vi "Station.Execution.vi"() -> ()   [LabVIEW 2015]
uses:
  Types/Main.StateVariables.ctl
  <vilib>/Utility/miscctls.llb/LVPositionTypeDef.ctl
  Types/Execute.UserEventRefs.ctl
  <vilib>/NI Veristand/Execution/Workspace/SystemStateRegEventRef.ctl
  <vilib>/NI Veristand/Execution/Workspace/Target State Info.ctl
  <vilib>/NI Veristand/Execution/Workspace/Target State.ctl
  <vilib>/NI Veristand/Execution/WaveformStreaming/Waveform Data Watcher Event Data (DBL).ctl
  <vilib>/NI Veristand/Execution/WaveformStreaming/WaveformStreamSpecification.ctl
  <vilib>/NI Veristand/Execution/Workspace/SystemStateEventRef.ctl
  <vilib>/NI Veristand/Execution/Workspace/WorkspaceAPI.ctl
  Types/UI.Object.ctl
  Types/Waveforms.Info.ctl
  <vilib>/NI Veristand/Execution/WaveformStreaming/Registered Waveform Streams Data Event Refnum (DBL).ctl
  <vilib>/NI Veristand/Execution/WaveformStreaming/WaveformDataWatcherDBL.ctl
  <vilib>/NI Veristand/Execution/WaveformStreaming/WaveformStreamingAPI.ctl
  <vilib>/NI/AMC/Read Termination Message.vi
  <vilib>/NI/AMC/Create Single Message.vi
  <vilib>/NI/AMC/Update Message Routing Info.vi
  <vilib>/NI/AMC/Create Multiple Messages.vi
  <vilib>/NI/AMC/Globals.vi
  <vilib>/NI/AMC/Send Message.vi
  NationalInstruments.VeriStand.ClientAPI
  <vilib>/NI Veristand/Execution/Workspace/NI_VS Workspace ExecutionAPI.lvlib
  <vilib>/NI/AMC/AMC.lvlib
  <vilib>/NI Veristand/Execution/WaveformStreaming/NI_VS Waveform Streaming Interface.lvlib
panel:
  in  "Tabs":string[](array[string])=["CAN.Fault Status", "CAN.IDH", "CAN.IDL", "CAN.LIN", "CAN.ODH", "CAN.ODL", "CAN.OPH", "DAQ.IDH", "DAQ.IDL", "DAQ.ODH", "DAQ.ODL", "DAQ.OPH"]
  in  "Station.ID":string="DUT1"
  out "Station ID":string="Station 1"
  in  "NIVS.Gateway IP Address":string="localhost"
  in  "NIVS.Workspace Event":refnum<event-registration>
  in  "ToolTab":enum32{"Enable", "Disable"}(tab)
  in  "Back":bool
  in  "Next":bool
  in  "Displays":enum32{"Default", "OSCOPE"}(tab)
  out "Table":string[][](table) caption="DMM"
  in  "Show Chart":bool
  out "Chart":dbl[][](graph)
  in  "Chart.Select":bool
  in  "Waveform.Select":bool
  out "Waveform.Graph":waveform(dbl)[](graph)
  in  "Waveform.Groups":u8(ring) items=["", "All"]
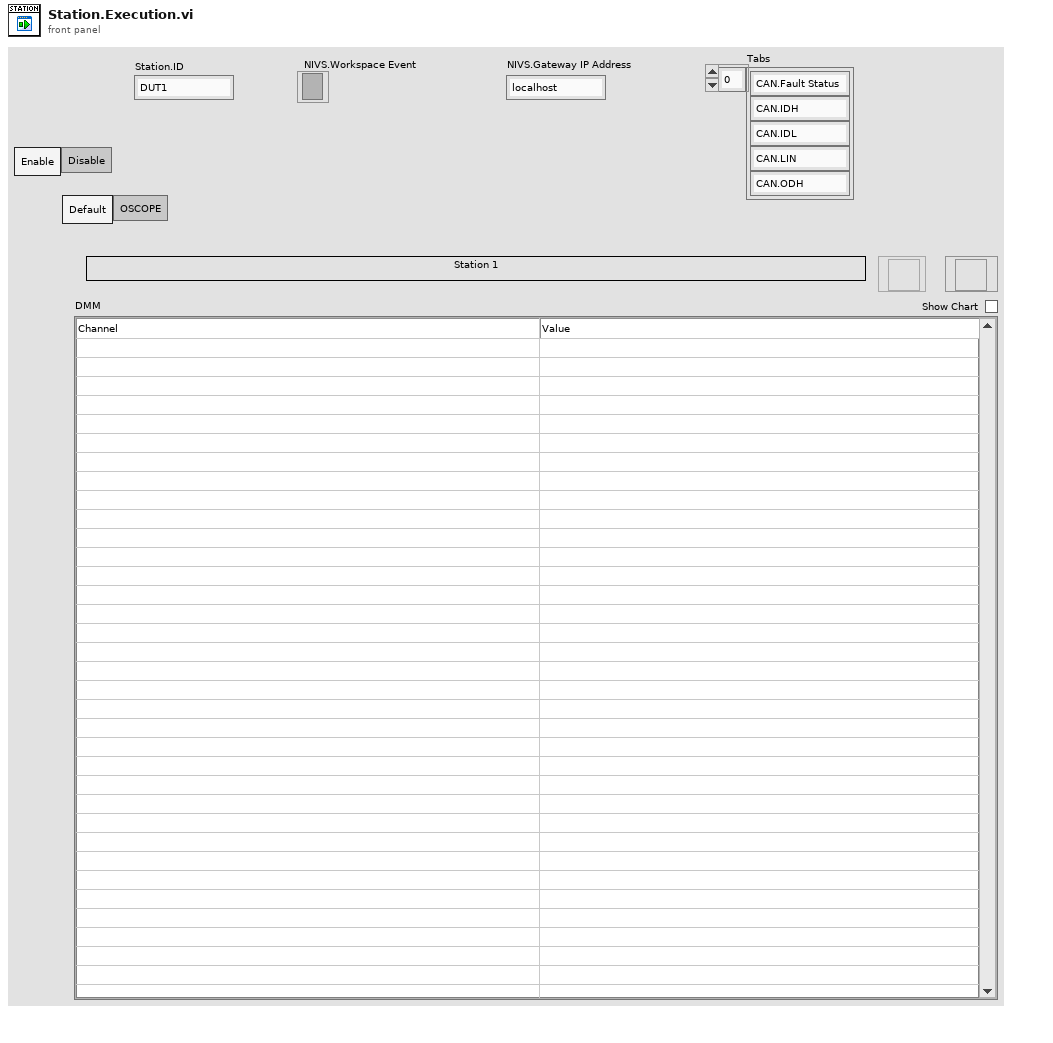
[diagram p1: front panel]
types:
  T1 = typedef "UI.Object.ctl" = cluster{"Name":string, "Paths":string[], "Names":string[], "Found?":bool}
  T2 = typedef "Main.StateVariables.ctl" = cluster{"Chart.Legend":T3, "Chart.Select":refnum<vi>, "Chart.Size":i32, "NIVS.Deployed":bool, "NIVS.Events":T4, "NIVS.GatewayIPAddress":string, "NIVS.SystemDefinitionFile":path, "NIVS.SystemStateRefs":T6, "NIVS.WorkspaceManager":T7, "NIVS.Open":bool, "Page.Index":u32, "Station.ID":string, "UI.Back":refnum<vi>, "UI.Next":refnum<vi>, "UI.Displays":refnum<vi>, "UI.ToolTab":refnum<vi>, "UI.Chart":refnum<vi>, "UI.ShowChart":bool, "UI.Table":refnum<vi>, "UI.Pages":T1[], "VI.Ref":refnum<vi>, "Waveform.Groups":refnum<vi>, "Waveform.Select":refnum<vi>, "Waveform.Graph":refnum<vi>, "Waveforms.Info":T8[], "Waveforms":cluster{"Refs":T9[], "Event.Refs":T10, "Streaming.Ref":T12}, "Waveforms.Reset":bool, "Waveforms.Size":i32, "Waveform.Legend":T3}
  T3 = typedef "LVPositionTypeDef.ctl" = cluster{"Left":i32, "Top":i32}
  T4 = typedef "Execute.UserEventRefs.ctl" = cluster{"SystemChangeEvent":T5, "WorkspaceEvent":refnum<event-registration>, "WaveformEvent":refnum<event-registration>}
  T5 = typedef "NI_VS Workspace ExecutionAPI.lvlib/SystemStateRegEventRef.ctl" = refnum<event-registration>
  T6 = typedef "NI_VS Workspace ExecutionAPI.lvlib/SystemStateEventRef.ctl" = cluster{"CustDatRef":refnum<user-event>, "EvtRef":refnum<k27>, "Target State User Event":refnum<user-event>}
  T7 = typedef "NI_VS Workspace ExecutionAPI.lvlib/WorkspaceAPI.ctl" = refnum<k24>
  T8 = typedef "Waveforms.Info.ctl" = cluster{"Name":string, "Path":string}
  T9 = typedef "NI_VS Waveform Streaming Interface.lvlib/WaveformStreamSpecification.ctl" = refnum<k24>
  T10 = typedef "NI_VS Waveform Streaming Interface.lvlib/Registered Waveform Streams Data Event Refnum (DBL).ctl" = cluster{"Callback Refnum":refnum<k27>, "Data Event":refnum<user-event>, "Event Refnum":refnum<event-registration>, "WaveformDataWatcherDBL":T11}
  T11 = typedef "NI_VS Waveform Streaming Interface.lvlib/WaveformDataWatcherDBL.ctl" = refnum<k24>
  T12 = typedef "NI_VS Waveform Streaming Interface.lvlib/WaveformStreamingAPI.ctl" = refnum<k24>
  T13 = typedef "AMC.lvlib/Message Queue.ctl" = refnum<queue>
  T14 = cluster{"Waveform.Refs":T9[], "WaveformStreaming.Event.Refs":T10, "WaveformStreaming.Ref":T12}
  T15 = typedef "AMC.lvlib/Message.ctl" = cluster{"name":string, "value":string, "attributes":T16, "receiver host":string, "receiver process":string, "source host":string, "source process":string, "priority message":bool, "acknowledge message":bool}
  T16 = typedef "Tools_KeyedArray.lvlib/KeyedArray.ctl" = cluster{"keys":string[], "values":string[]}
  T17 = typedef "LVPoint32TypeDef.ctl" = cluster{"Horizontal":i32, "Vertical":i32}
  T18 = cluster{"Refs":T9[], "Event.Refs":T10, "Streaming.Ref":T12}
  T19 = typedef "NI_VS Workspace ExecutionAPI.lvlib/SystemState.ctl" = u8
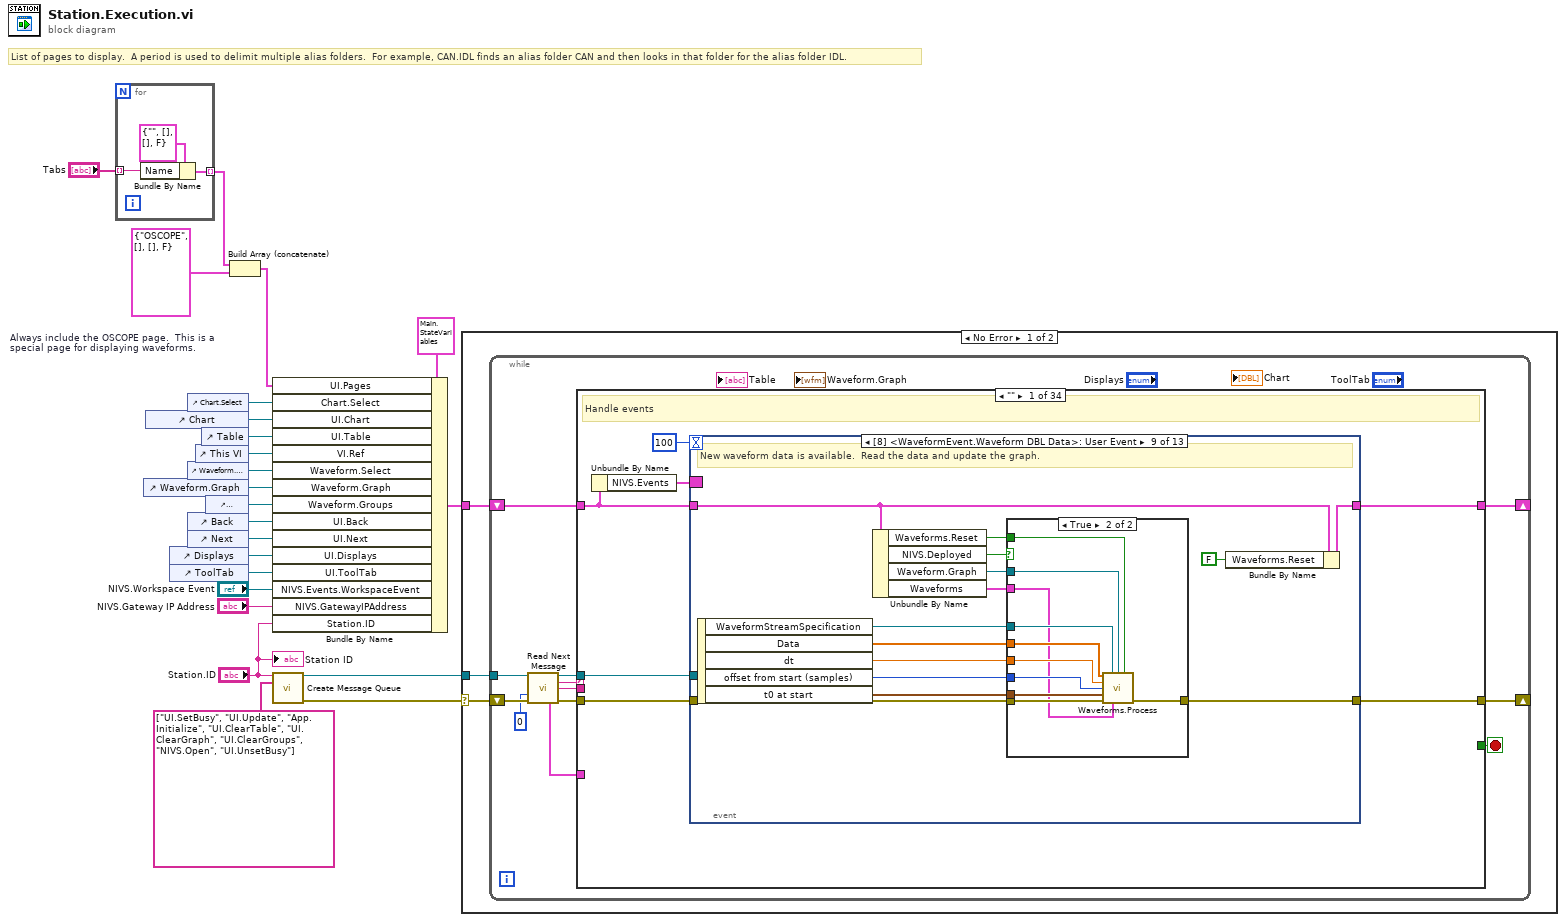
[diagram p0: block diagram]
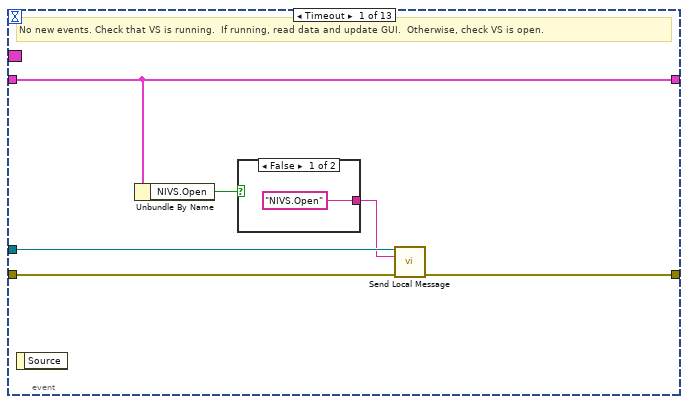
[diagram p2: hidden frame]
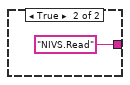
[diagram p3: hidden frame]
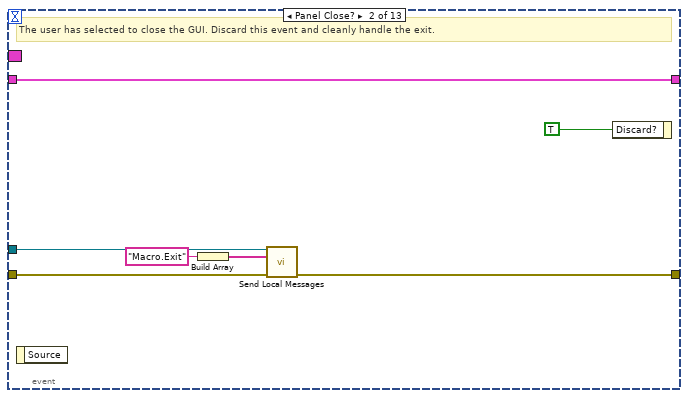
[diagram p4: hidden frame]
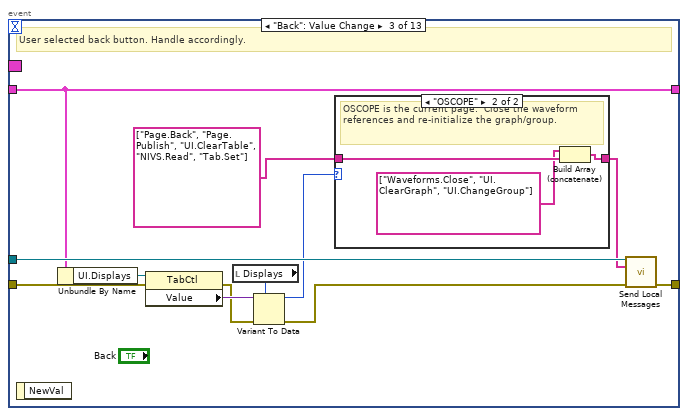
[diagram p5: hidden frame]
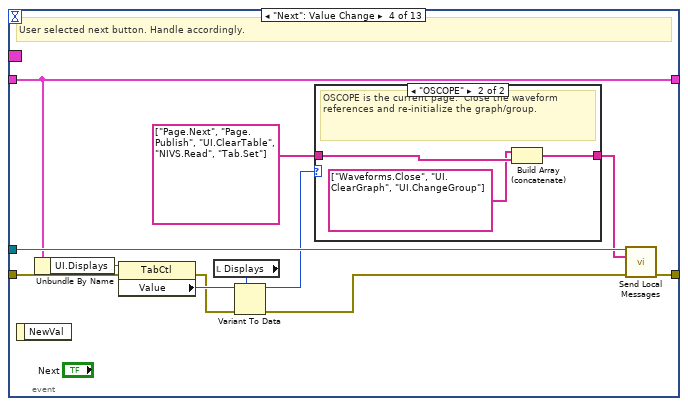
[diagram p7: hidden frame]
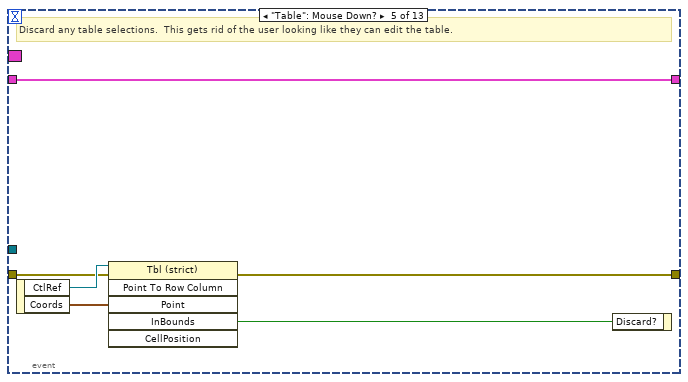
[diagram p9: hidden frame]
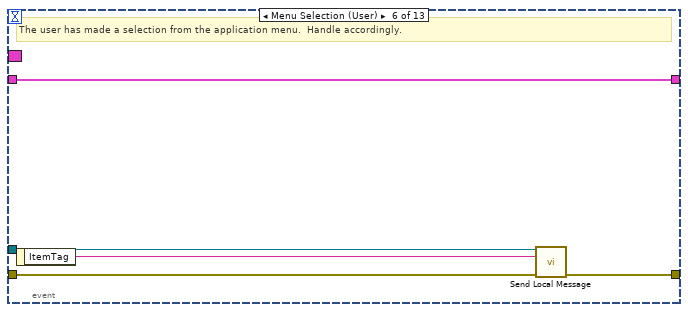
[diagram p10: hidden frame]
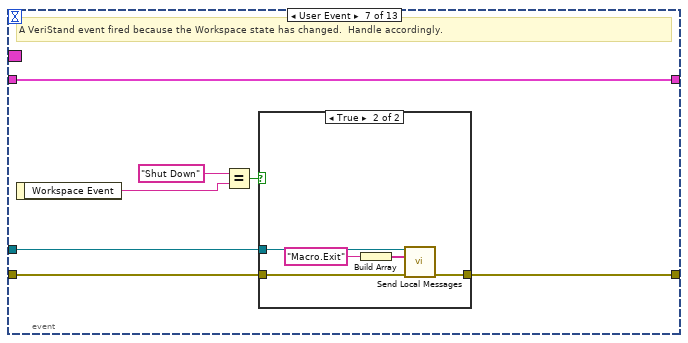
[diagram p11: hidden frame]
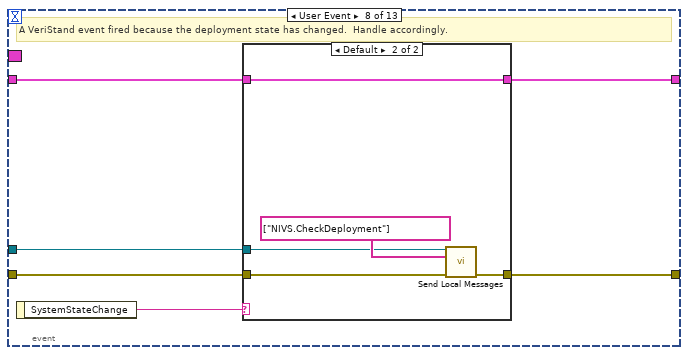
[diagram p13: hidden frame]
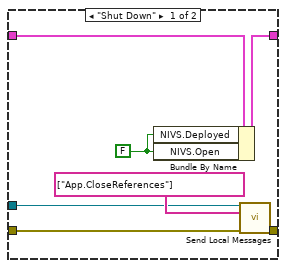
[diagram p14: hidden frame]
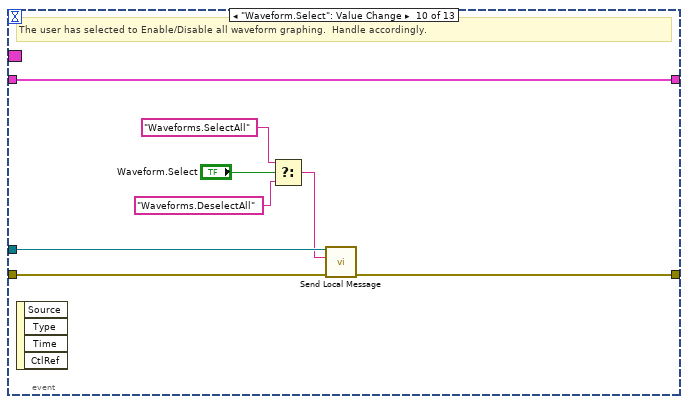
[diagram p16: hidden frame]
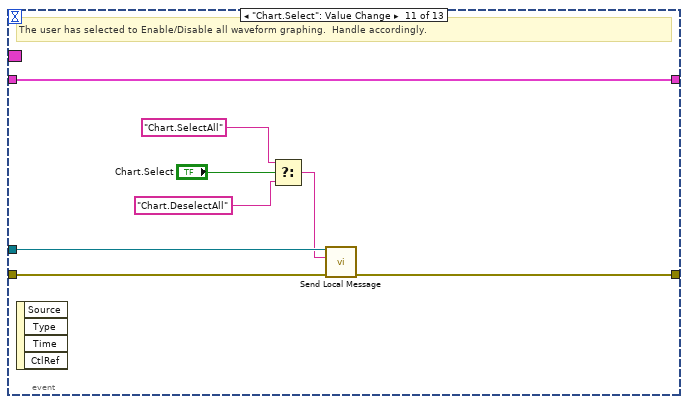
[diagram p17: hidden frame]
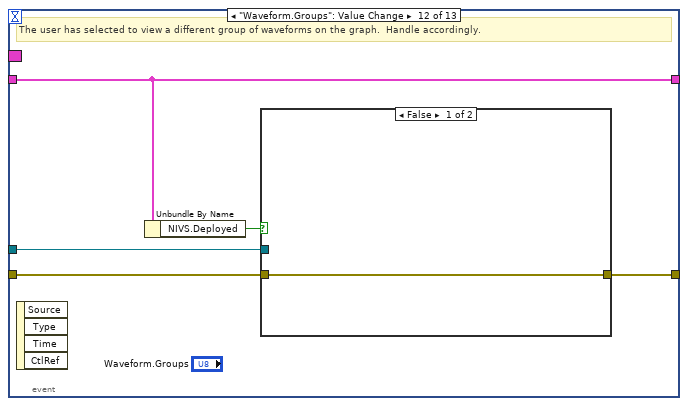
[diagram p18: hidden frame]
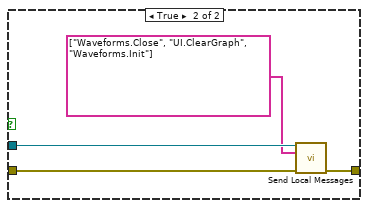
[diagram p19: hidden frame]
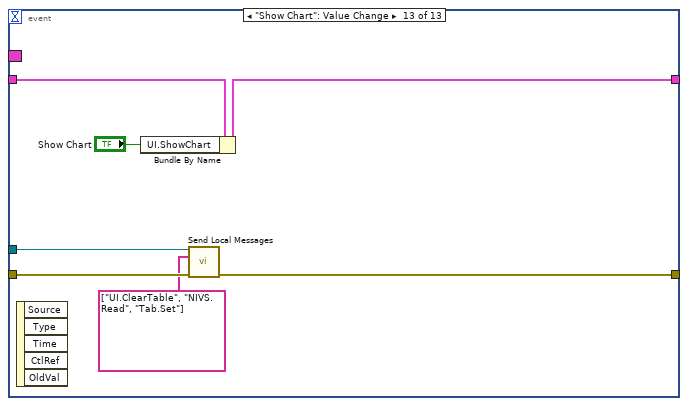
[diagram p20: hidden frame]
diagram:
  w5 = T1 {"Name"="OSCOPE", "Paths"=[], "Names"=[], "Found?"=FALSE}  # Always include the OSCOPE page.  This is a special page for displaying waveforms.
  # "List of pages to display.  A period is used to delimit multiple alias folders.  For example, CAN.IDL finds an alias folder CAN and then looks in that folder for the alias folder IDL."
  n1 = for {
    tunnel: "Tabs" -> [w25] mode=indexing
    tunnel: [w24] -> w4 mode=indexing
    n2 = Bundle By Name(cluster=T1 {"Name"="", "Paths"=[], "Names"=[], "Found?"=FALSE} ("Table"), "Name"=w25) -> (w24:T1)
  }
  n3 = control-ref of="Waveform.Graph"() -> (w8:refnum<vi>)
  n4 = control-ref of="Chart"() -> (w2:refnum<vi>)
  n5 = control-ref of="Displays"() -> (w12:refnum<vi>)
  n6 = control-ref of="ToolTab"() -> (w18:refnum<vi>)
  n7 = control-ref of="Chart.Select"() -> (w1:refnum<vi>)
  n8 = control-ref of="Waveform.Select"() -> (w9:refnum<vi>)
  n9 = control-ref of="Back"() -> (w16:refnum<vi>)
  n10 = control-ref of="Next"() -> (w17:refnum<vi>)
  n11 = control-ref of="This VI"() -> (w11:refnum<vi>)
  n12 = control-ref of="Table"() -> (w3:refnum<vi>)
  n13 = control-ref of="Waveform.Groups"() -> (w10:refnum<vi>)
  n14 = Build Array (concatenate)(w4, w5) -> (w6:T1[])
  n15 = Bundle By Name(cluster=T2 {"Chart.Legend"={"Left"=0, "Top"=0}, "Chart.Select"=refnum, "Chart.Size"=0, "NIVS.Deployed"=FALSE, "NIVS.Events"={"SystemChangeEvent"=refnum, "WorkspaceEvent"=refnum, "WaveformEvent"=refnum}, "NIVS.GatewayIPAddress"="", "NIVS.SystemDefinitionFile"=path "", "NIVS.SystemStateRefs"={"CustDatRef"=refnum, "EvtRef"=refnum, "Target State User Event"=refnum}, "NIVS.WorkspaceManager"=refnum, "NIVS.Open"=FALSE, "Page.Index"=0, "Station.ID"="", "UI.Back"=refnum, "UI.Next"=refnum, "UI.Displays"=refnum, "UI.ToolTab"=refnum, "UI.Chart"=refnum, "UI.ShowChart"=FALSE, "UI.Table"=refnum, "UI.Pages"=[], "VI.Ref"=refnum, "Waveform.Groups"=refnum, "Waveform.Select"=refnum, "Waveform.Graph"=refnum, "Waveforms.Info"=[], "Waveforms"={"Refs"=[], "Event.Refs"={"Callback Refnum"=refnum, "Data Event"=refnum, "Event Refnum"=refnum, "WaveformDataWatcherDBL"=refnum}, "Streaming.Ref"=refnum}, "Waveforms.Reset"=FALSE, "Waveforms.Size"=0, "Waveform.Legend"={"Left"=0, "Top"=0}} ("State Variables"), "UI.Pages"=w6, "Chart.Select"=w1, "UI.Chart"=w2, "UI.Table"=w3, "VI.Ref"=w11, "Waveform.Select"=w9, "Waveform.Graph"=w8, "Waveform.Groups"=w10, "UI.Back"=w16, "UI.Next"=w17, "UI.Displays"=w12, "UI.ToolTab"=w18, "NIVS.Events.WorkspaceEvent"="NIVS.Workspace Event", "NIVS.GatewayIPAddress"="NIVS.Gateway IP Address", "Station.ID"="Station.ID") -> (w23:T2)
  n16 = call <vilib>:"Create Message Queue.vi"("message queue name"="Station.ID", "initial message names"=string[] ["UI.SetBusy", "UI.Update", "App.Initialize", "UI.ClearTable", "UI.ClearGraph", "UI.ClearGroups", "NIVS.Open", "UI.UnsetBusy"]) -> ("message queue out"=w20:T13, "error out"=w13:errorcluster)  [unwired: 12 in]
  n17 = case shown="No Error" w13 {
    selector: w13 -> [w27 _]
    tunnel: w23 -> [w28 _]
    tunnel: w20 -> [w29 _]
    frame No Error {
      n18 = while {
        shift-right: [w40] -> _
        shift-left: w28 -> [w41]
        shift-right: [w30] -> _
        shift-left: w27 -> [w39]
        tunnel: w29 -> [w37]
        stop <- w38 stop-if-true
        n19 = call <vilib>:"Read Next Message.vi"("message queue in"=w37, "timeout (1 ms)"=0 ("Timeout"), "error in"=w39) -> ("message queue out"=w34:T13, "message name"=w33:string, "message value"=w32:string, "message"=w31:T15, "error out"=w35:errorcluster)  [unwired: 5 in, 3 out]
        n20 = case shown="\"\"" w33 {
          selector: w33 -> [_ _ _ _ _ _ _ _ _ _ _ _ _ _ _ _ _ _ _ _ _ w416 w422 _ _ _ _ _ _ _ _ _ _ _]
          tunnel: w41 -> [w44 w198 w202 w211 w220 w237 w259 w272 w287 w291 w310 w338 w342 w344 w348 w362 w375 w383 w404 w409 w411 w420 w425 w433 w438 w441 w444 w447 w465 w468 w482 w504 w516 w524]
          tunnel: [w48 w197 w203 w210 w220 w237 w259 w272 w287 w290 w309 w336 w342 w343 w347 w362 w375 w382 w403 w409 w410 w420 w425 w433 w438 w441 w444 w446 w465 w467 w482 w504 w515 w524] -> w40
          tunnel: [w45 w199 w205 w212 w221 w231 w253 w276 w285 w297 w311 w337 w340 w346 w350 w351 w368 w396 w406 w407 w412 w417 w421 w426 w435 w439 w442 w458 w462 w469 w476 w498 w514 w523] -> w30
          tunnel: w35 -> [w46 w200 w204 w212 w222 w233 w255 w275 w286 w292 w312 w339 w341 w345 w349 w351 w369 w388 w405 w408 w412 w417 w421 w427 w436 w440 w443 w453 w463 w466 w478 w500 w519 w523]
          tunnel: [_ _ _ _ TRUE _ _ _ _ _ _ _ _ _ _ _ _ _ _ _ _ _ _ _ _ _ _ _ _ _ _ _ _ _] -> w38
          tunnel: w34 -> [w42 _ _ _ w223 _ _ w273 w284 w296 w308 _ _ _ _ _ _ w386 _ _ _ _ _ _ _ _ _ _ _ _ _ _ _ _]
          tunnel: w32 -> [_ _ _ _ _ _ _ _ _ _ _ _ _ _ _ _ _ w397 _ _ _ _ _ _ _ _ _ _ _ _ _ _ _ _]
          tunnel: w31 -> [_ _ _ _ _ _ _ _ _ _ _ _ _ _ _ _ _ _ _ _ _ _ _ _ _ _ _ _ _ _ _ _ _ _]
          frame "" {
            # "Handle events"
            n21 = Unbundle By Name(w44) -> ("NIVS.Events"=w43:T4)
            n22 = event shown="[8] <WaveformEvent.Waveform DBL Data>: User Event" {
              selector: w43 -> [_ _ _ _ _ _ _ _ _ _ _ _ _]
              dyn-events: _ -> [_ _ _ _ _ _ _ _ _ _ _ _ _]
              timeout: 100 -> [_ _ _ _ _ _ _ _ _ _ _ _ _]
              tunnel: [w50 w62 w71 w89 w101 w102 w111 w120 w139 w170 w178 w180 w193] -> w48
              tunnel: w44 -> [w50 w62 w71 w89 w101 w102 w111 w121 w140 w170 w178 w180 w194]
              tunnel: [w52 w59 w75 w91 w96 w105 w109 w122 w150 w168 w176 w182 w191] -> w45
              tunnel: w46 -> [w53 w60 w69 w87 w98 w106 w110 w125 w151 w169 w177 w183 w192]
              tunnel: w42 -> [w54 w58 w74 w90 _ w104 w108 w124 _ w167 w175 w181 w190]
              event Timeout {
                # "No new events. Check that VS is running.  If running, read data and update GUI.  Otherwise, check VS is open."
                n23 = event-data() -> ()  [unwired: 1 in, 1 out]
                n24 = Unbundle By Name(w50) -> ("NIVS.Open"=w49:bool)
                n25 = case shown="False" w49 {
                  tunnel: ["NIVS.Open" ("message name") "NIVS.Read" ("message name")] -> w51
                  frame False {
                  }
                  frame True {
                  }
                }
                n26 = call <vilib>:"Send Local Message.vi"("message queue in"=w54, "message name"=w51, "error in"=w53) -> ("error out"=w52:errorcluster)  [unwired: 10 in, 2 out]
              }
              event Panel Close? {
                # "The user has selected to close the GUI. Discard this event and cleanly handle the exit."
                n27 = event-data() -> ()  [unwired: 1 in, 1 out]
                n28 = Build Array("Macro.Exit") -> (w57:string[])
                n29 = call <vilib>:"Send Local Messages.vi"("message queue in"=w58, "message names"=w57, "error in"=w60) -> ("error out"=w59:errorcluster)  [unwired: 10 in, 2 out]
                n30 = event-data("Discard?"=TRUE) -> ()  [unwired: 1 in, 1 out]
              }
              event "Back": Value Change {
                # "User selected back button. Handle accordingly."
                n31 = event-data() -> ()  [unwired: 1 in, 1 out]
                n32 = Unbundle By Name(w71) -> ("UI.Displays"=w70:refnum<vi>)
                n33 = property class="TabCtl"(reference=w70, error in=w69) -> (error out=w67:errorcluster, "Value"=w68:variant)  [unwired: 1 out]
                n34 = local read "Displays"() -> (w65:enum32{"Default", "OSCOPE"})
                n35 = Variant To Data(error in=w67, type=w65, Variant=w68) -> (data=w64:enum32{"Default", "OSCOPE"}, error out=w66:errorcluster)
                n36 = case shown="\"OSCOPE\"" w64 {
                  tunnel: [w76 w78] -> w73
                  tunnel: string[] ["Page.Back", "Page.Publish", "UI.ClearTable", "NIVS.Read", "Tab.Set"] ("message names") -> [w76 w79]
                  frame Default {
                    # "Do nothing extra."
                  }
                  frame "OSCOPE" {
                    # "OSCOPE is the current page.  Close the waveform references and re-initialize the graph/group."
                    n37 = Build Array (concatenate)(string[] ["Waveforms.Close", "UI.ClearGraph", "UI.ChangeGroup"], w79) -> (w78:string[])
                  }
                }
                n38 = call <vilib>:"Send Local Messages.vi"("message queue in"=w74, "message names"=w73, "error in"=w66) -> ("error out"=w75:errorcluster)  [unwired: 10 in, 2 out]
              }
              event "Next": Value Change {
                # "User selected next button. Handle accordingly."
                n39 = event-data() -> ()  [unwired: 1 in, 1 out]
                n40 = Unbundle By Name(w89) -> ("UI.Displays"=w88:refnum<vi>)
                n41 = property class="TabCtl"(reference=w88, error in=w87) -> (error out=w83:errorcluster, "Value"=w84:variant)  [unwired: 1 out]
                n42 = local read "Displays"() -> (w81:enum32{"Default", "OSCOPE"})
                n43 = Variant To Data(error in=w83, type=w81, Variant=w84) -> (data=w80:enum32{"Default", "OSCOPE"}, error out=w82:errorcluster)
                n44 = case shown="\"OSCOPE\"" w80 {
                  tunnel: [w92 w94] -> w85
                  tunnel: string[] ["Page.Next", "Page.Publish", "UI.ClearTable", "NIVS.Read", "Tab.Set"] ("message names") -> [w92 w95]
                  frame Default {
                    # "Do nothing extra."
                  }
                  frame "OSCOPE" {
                    # "OSCOPE is the current page.  Close the waveform references and re-initialize the graph/group."
                    n45 = Build Array (concatenate)(string[] ["Waveforms.Close", "UI.ClearGraph", "UI.ChangeGroup"], w95) -> (w94:string[])
                  }
                }
                n46 = call <vilib>:"Send Local Messages.vi"("message queue in"=w90, "message names"=w85, "error in"=w82) -> ("error out"=w91:errorcluster)  [unwired: 10 in, 2 out]
              }
              event "Table": Mouse Down? {
                # "Discard any table selections.  This gets rid of the user looking like they can edit the table."
                n47 = event-data() -> ("CtlRef"=w100:refnum<vi>, "Coords"=w99:T17)  [unwired: 1 in]
                n48 = invoke class="Tbl (strict)" method="Point To Row Column"(reference=w100, error in=w98, "Point"=w99) -> (error out=w96:errorcluster, "InBounds"=w97:bool)  [unwired: 3 in, 4 out]
                n49 = event-data("Discard?"=w97) -> ()  [unwired: 1 in, 1 out]
              }
              event Menu Selection (User) {
                # "The user has made a selection from the application menu.  Handle accordingly."
                n50 = event-data() -> ("ItemTag"=w103:string)  [unwired: 1 in]
                n51 = call <vilib>:"Send Local Message.vi"("message queue in"=w104, "message name"=w103, "error in"=w106) -> ("error out"=w105:errorcluster)  [unwired: 10 in, 2 out]
              }
              event User Event {
                # "A VeriStand event fired because the Workspace state has changed.  Handle accordingly."
                n52 = event-data() -> ("Workspace Event"=w107:string)  [unwired: 1 in]
                n53 = Equal?(x="Shut Down" ("y"), y=w107) -> (x = y?=w112:bool)
                n54 = case shown="True" w112 {
                  tunnel: w110 -> [w114 w119]
                  tunnel: [w114 w118] -> w109
                  tunnel: w108 -> [_ w117]
                  frame False {
                  }
                  frame True {
                    n55 = Build Array("Macro.Exit" ("y")) -> (w116:string[])
                    n56 = call <vilib>:"Send Local Messages.vi"("message queue in"=w117, "message names"=w116, "error in"=w119) -> ("error out"=w118:errorcluster)  [unwired: 10 in, 2 out]
                  }
                }
              }
              event User Event {
                # "A VeriStand event fired because the deployment state has changed.  Handle accordingly."
                n57 = event-data() -> ("SystemStateChange"=w123:string)  [unwired: 1 in]
                n58 = case shown="Default" w123 {
                  tunnel: w125 -> [w131 w136]
                  tunnel: w124 -> [w130 w135]
                  tunnel: [w129 w134] -> w122
                  tunnel: w121 -> [w128 w133]
                  tunnel: [w127 w133] -> w120
                  frame "Shut Down" {
                    w126 = FALSE ("NIVS.Open")
                    n59 = Bundle By Name(cluster=w128, "NIVS.Deployed"=w126, "NIVS.Open"=w126) -> (w127:T2)
                    n60 = call <vilib>:"Send Local Messages.vi"("message queue in"=w130, "message names"=string[] ["App.CloseReferences"], "error in"=w131) -> ("error out"=w129:errorcluster)  [unwired: 10 in, 2 out]
                  }
                  frame Default {
                    n61 = call <vilib>:"Send Local Messages.vi"("message queue in"=w135, "message names"=string[] ["NIVS.CheckDeployment"], "error in"=w136) -> ("error out"=w134:errorcluster)  [unwired: 10 in, 2 out]
                  }
                }
              }
              event User Event {
                # "New waveform data is available.  Read the data and update the graph."
                n62 = event-data() -> ("WaveformStreamSpecification"=w149:T9, "Data"=w147:dbl[], "dt"=w146:dbl, "offset from start (samples)"=w145:u64, "t0 at start"=w144:timestamp)  [unwired: 1 in]
                n63 = Unbundle By Name(w140) -> ("Waveforms.Reset"=w141:bool, "NIVS.Deployed"=w142:bool, "Waveform.Graph"=w148:refnum<vi>, "Waveforms"=w143:T18)
                n64 = case shown="True" w142 {
                  tunnel: w151 -> [w152 w162]
                  tunnel: [w152 w161] -> w150
                  tunnel: w149 -> [_ w160]
                  tunnel: w148 -> [_ w159]
                  tunnel: w147 -> [_ w158]
                  tunnel: w146 -> [_ w157]
                  tunnel: w145 -> [_ w156]
                  tunnel: w144 -> [_ w155]
                  tunnel: w143 -> [_ w154]
                  tunnel: w141 -> [_ w153]
                  frame False {
                  }
                  frame True {
                    n65 = call "Waveforms.Process.vi"("Data"=w158, "Waveform.Ref"=w160, "WaveformGraph.Ref"=w159, "Reset?"=w153, "dt"=w157, "offset from start (samples)"=w156, "t0 at start"=w155, "error in (no error)"=w162, "Waveforms"=w154) -> ("error out"=w161:errorcluster)  [unwired: 6 in]
                  }
                }
                n66 = Bundle By Name(cluster=w140, "Waveforms.Reset"=FALSE) -> (w139:T2)
              }
              event "Waveform.Select": Value Change {
                # "The user has selected to Enable/Disable all waveform graphing.  Handle accordingly."
                n67 = event-data() -> ()  [unwired: 1 in, 4 out]
                n68 = Select(t="Waveforms.SelectAll", s="Waveform.Select", f="Waveforms.DeselectAll") -> (s? t:f=w163:string)
                n69 = call <vilib>:"Send Local Message.vi"("message queue in"=w167, "message name"=w163, "error in"=w169) -> ("error out"=w168:errorcluster)  [unwired: 10 in, 2 out]
              }
              event "Chart.Select": Value Change {
                # "The user has selected to Enable/Disable all waveform graphing.  Handle accordingly."
                n70 = event-data() -> ()  [unwired: 1 in, 4 out]
                n71 = Select(t="Chart.SelectAll", s="Chart.Select", f="Chart.DeselectAll") -> (s? t:f=w172:string)
                n72 = call <vilib>:"Send Local Message.vi"("message queue in"=w175, "message name"=w172, "error in"=w177) -> ("error out"=w176:errorcluster)  [unwired: 10 in, 2 out]
              }
              event "Waveform.Groups": Value Change {
                # "The user has selected to view a different group of waveforms on the graph.  Handle accordingly."
                n73 = event-data() -> ()  [unwired: 1 in, 4 out]
                n74 = Unbundle By Name(w180) -> ("NIVS.Deployed"=w179:bool)
                n75 = case shown="False" w179 {
                  tunnel: w183 -> [w184 w188]
                  tunnel: [w184 w187] -> w182
                  tunnel: w181 -> [_ w186]
                  frame False {
                  }
                  frame True {
                    n76 = call <vilib>:"Send Local Messages.vi"("message queue in"=w186, "message names"=string[] ["Waveforms.Close", "UI.ClearGraph", "Waveforms.Init"], "error in"=w188) -> ("error out"=w187:errorcluster)  [unwired: 10 in, 2 out]
                  }
                }
              }
              event "Show Chart": Value Change {
                n77 = event-data() -> ()  [unwired: 1 in, 5 out]
                n78 = Bundle By Name(cluster=w194, "UI.ShowChart"="Show Chart") -> (w193:T2)
                n79 = call <vilib>:"Send Local Messages.vi"("message queue in"=w190, "message names"=string[] ["UI.ClearTable", "NIVS.Read", "Tab.Set"], "error in"=w192) -> ("error out"=w191:errorcluster)  [unwired: 10 in, 2 out]
              }
            }
          }
          frame "App.Initialize" {
            # "Initialize the GUI."
            n80 = call "Execute.Initialize.vi"("error in (no error)"=w200, "State Variables"=w198) -> ("error out"=w199:errorcluster, "State Variables"=w197:T2)  [unwired: 8 in]
            n81 = local write "Show Chart"(FALSE ("Show Chart")) -> ()
          }
          frame "App.CreateEvents" {
            # "Get events to stay in sync with the VeriStand deployment state."
            n82 = Unbundle By Name(w202) -> ("NIVS.WorkspaceManager"=w206:T7)
            n83 = call <vilib>:"NI VeriStand - Open Engine State Change Notification.vi"("error in (no error)"=w204, "WorkspaceManager in"=w206) -> ("error out"=w205:errorcluster, "SystemStateRefs"=w208:T6, "SystemChangeEventRef"=w207:T5, "WorkspaceManager out"=w201:T7)  [unwired: 6 in]
            n84 = Bundle By Name(cluster=w202, "NIVS.WorkspaceManager"=w201, "NIVS.Events.SystemChangeEvent"=w207, "NIVS.SystemStateRefs"=w208) -> (w203:T2)
          }
          frame "App.CloseReferences" {
            w209 = FALSE ("NIVS.Open")
            # "Close all the reference to VeriStand."
            n85 = flat-sequence {
              tunnel: w211 -> [w216]
              tunnel: [w215] -> _
              tunnel: [w214] -> _
              tunnel: [w213] -> _
              frame #0 {
                n86 = Unbundle By Name(w216) -> ("NIVS.Events"=w217:T4, "NIVS.SystemStateRefs"=w219:T6, "NIVS.WorkspaceManager"=w218:T7)
                n87 = call <vilib>:"NI VeriStand - Close Workspace Manager Reference.vi"("WorkspaceManager"=w218) -> ("error out"=w213:errorcluster)  [unwired: 10 in]
                n88 = call <vilib>:"NI VeriStand - Close Engine State Change Notification.vi"("SystemStateRefs"=w219) -> ("error out"=w214:errorcluster)  [unwired: 10 in]
                n89 = Unregister For Events(event registration refnum=w217) -> (error out=w215:errorcluster)  [unwired: 1 in]
              }
            }
            n90 = Bundle By Name(cluster=w211, "NIVS.Open"=w209, "NIVS.Deployed"=w209) -> (w210:T2)
          }
          frame "App.Exit" {
            # "Exit the application."
            n91 = call <vilib>:"Destroy Message Queue.vi"("message queue in"=w223, "error in"=w222) -> ("error out"=w221:errorcluster)  [unwired: 11 in, 2 out]
          }
          frame "Chart.SelectAll" {
            # "Enable all the channels on the graph."
            n92 = Unbundle By Name(w237) -> ("Chart.Size"=w225:i32, "UI.Chart"=w226:refnum<vi>, "VI.Ref"=w236:refnum<vi>)
            n93 = property class="VI"(reference=w236, error in=w233) -> (error out=w234:errorcluster, "Panel"=w235:refnum<vi>)  [unwired: 1 out]
            n94 = property class="Pnl"(reference=w235, error in=w234, "DeferPanUpdts"=TRUE ("Defer Panel Updates")) -> (reference out=w229:refnum<vi>, error out=w227:errorcluster)
            n95 = for {
              N: w225 -> [_]
              tunnel: w226 -> [w246]
              shift-right: [w242] -> w230
              shift-left: w227 -> [w245]
              i -> [w244]
              n96 = property class="WFChart (strict)"(reference=w246, error in=w245, "Active Plot"=w244, "Plot.Visible?"=TRUE ("Legend:Visible")) -> (error out=w242:errorcluster)  [unwired: 1 out]
            }
            n97 = flat-sequence {
              tunnel: [w241] -> w231
              tunnel: w230 -> [w241]
              tunnel: w229 -> [w240]
              tunnel: FALSE ("Defer Panel Updates") -> [w239]
              tunnel: [w238] -> _
              frame #0 {
                n98 = property class="Pnl"(reference=w240, "DeferPanUpdts"=w239) -> (error out=w238:errorcluster)  [unwired: 1 in, 1 out]
              }
            }
          }
          frame "Chart.DeselectAll" {
            # "Enable all the channels on the graph."
            n99 = Unbundle By Name(w259) -> ("Chart.Size"=w247:i32, "UI.Chart"=w248:refnum<vi>, "VI.Ref"=w258:refnum<vi>)
            n100 = property class="VI"(reference=w258, error in=w255) -> (error out=w256:errorcluster, "Panel"=w257:refnum<vi>)  [unwired: 1 out]
            n101 = property class="Pnl"(reference=w257, error in=w256, "DeferPanUpdts"=TRUE ("Defer Panel Updates")) -> (reference out=w251:refnum<vi>, error out=w249:errorcluster)
            n102 = for {
              N: w247 -> [_]
              tunnel: w248 -> [w268]
              shift-right: [w264] -> w252
              shift-left: w249 -> [w267]
              i -> [w266]
              n103 = property class="WFChart (strict)"(reference=w268, error in=w267, "Active Plot"=w266, "Plot.Visible?"=FALSE ("Legend:Visible")) -> (error out=w264:errorcluster)  [unwired: 1 out]
            }
            n104 = flat-sequence {
              tunnel: [w263] -> w253
              tunnel: w252 -> [w263]
              tunnel: w251 -> [w262]
              tunnel: FALSE ("Defer Panel Updates") -> [w261]
              tunnel: [w260] -> _
              frame #0 {
                n105 = property class="Pnl"(reference=w262, "DeferPanUpdts"=w261) -> (error out=w260:errorcluster)  [unwired: 1 in, 1 out]
              }
            }
          }
          frame "Error" {
            # "Clear any expected errors from VeriStand.  Handle any remaining errors.  Attempt to restart the application."
            n106 = for {
              shift-right: [w281] -> w270
              shift-left: w275 -> [w282]
              tunnel: i32[] [-307652, -307654] -> [w280] mode=indexing
              n107 = call <vilib>:"Clear Errors.vi"("error in (no error)"=w282, "specific error code to clear (0: all)"=w280) -> ("error out"=w281:errorcluster)  [unwired: 4 in, 1 out]
            }
            n108 = case shown="Error" w270 {
              selector: w270 -> [w277 w278]
              tunnel: [w277 w279] -> w271
              frame No Error {
              }
              frame Error {
                n109 = call <vilib>:"Clear Errors.vi"("error in (no error)"=w278) -> ("error out"=w279:errorcluster)  [unwired: 5 in, 1 out]
                n110 = call "Error.Display.vi"("error in (no error)"=w278) -> ()  [unwired: 11 in]
              }
            }
            n111 = call <vilib>:"Send Local Messages.vi"("message queue in"=w273, "message names"=string[] ["UI.SetBusy", "UI.Update", "Waveforms.Close", "UI.ClearGraph", "UI.ClearGroups", "App.CloseReferences", "App.Initialize", "UI.ClearTable", "NIVS.Open", "UI.UnsetBusy"], "error in"=w271) -> ("error out"=w276:errorcluster)  [unwired: 10 in, 2 out]
          }
          frame "Macro.Exit" {
            # "Queue up all the states required to exit the application cleanly."
            n112 = call <vilib>:"Send Local Messages.vi"("message queue in"=w284, "message names"=string[] ["Waveforms.Close", "App.CloseReferences", "UI.Close", "App.Exit"], "error in"=w286) -> ("error out"=w285:errorcluster)  [unwired: 10 in, 2 out]
          }
          frame "NIVS.CheckDeployment" {
            # "VeriStand is open. Check the project deployment state."
            n113 = Unbundle By Name(w291) -> ("NIVS.WorkspaceManager"=w294:T7)
            n114 = call <vilib>:"NI VeriStand - Get System State.vi"("error in (no error)"=w292, "WorkspaceManager in"=w294) -> ("error out"=w288:errorcluster, "System State"=w295:T19, "System Definition File"=w293:path)  [unwired: 5 in, 2 out]
            n115 = case shown="0, Default" w295 {
              tunnel: w291 -> [w302 w307]
              tunnel: [w301 w305] -> w290
              tunnel: w293 -> [_ w304]
              tunnel: [string[] ["Waveforms.Close", "UI.Update", "UI.ClearTable", "UI.ClearGraph", "UI.ClearGroups", "NIVS.GetChannels", "Pages.Publish"] string[] ["NIVS.GetChannels", "Pages.Publish", "App.Initialize", "UI.UpdateGroups", "UI.Update", "Tab.Set"]] -> w289
              frame 0, Default {
                # "Not Deployed."
                n116 = Bundle By Name(cluster=w302, "NIVS.Deployed"=FALSE ("Connected"), "NIVS.SystemDefinitionFile"=path "") -> (w301:T2)
              }
              frame 1 {
                # "Deployed."
                n117 = Bundle By Name(cluster=w307, "NIVS.Deployed"=TRUE ("Connected"), "NIVS.SystemDefinitionFile"=w304) -> (w305:T2)
              }
            }
            n118 = call <vilib>:"Send Local Messages.vi"("message queue in"=w296, "message names"=w289, "error in"=w288) -> ("error out"=w297:errorcluster)  [unwired: 10 in, 2 out]
          }
          frame "NIVS.Open" {
            # "Attempt to open a connection to VeriStand."
            n119 = Unbundle By Name(w310) -> ("NIVS.GatewayIPAddress"=w313:string)
            n120 = case shown="No Error" w312 {
              selector: w312 -> [w316 w334]
              tunnel: w313 -> [w321 _]
              tunnel: [w315 w334] -> w311
              tunnel: w310 -> [w319 w335]
              tunnel: [w317 w335] -> w309
              tunnel: w308 -> [w314 _]
              frame No Error {
                n121 = call <vilib>:"NI VeriStand - Open Workspace Manager Reference.vi"("Gateway IP Address (\"\": localhost)"=w321) -> ("error out"=w320:errorcluster, "WorkspaceManager"=w318:T7)  [unwired: 9 in]
                n122 = case shown="No Error" w320 {
                  tunnel: w319 -> [w329 w332]
                  tunnel: w318 -> [w328 _]
                  tunnel: [w326 w331] -> w317
                  tunnel: w316 -> [w325 w333]
                  tunnel: [w324 w333] -> w315
                  tunnel: w314 -> [w323 _]
                  frame No Error {
                    # "VeriStand is open and connected."
                    n123 = Bundle By Name(cluster=w329, "NIVS.Open"=TRUE, "NIVS.WorkspaceManager"=w328) -> (w326:T2)
                    n124 = call <vilib>:"Send Local Messages.vi"("message queue in"=w323, "message names"=string[] ["App.CreateEvents", "NIVS.CheckDeployment"], "error in"=w325) -> ("error out"=w324:errorcluster)  [unwired: 10 in, 2 out]
                  }
                  frame Error {
                    # "VeriStand is still not open."
                    n125 = Bundle By Name(cluster=w332, "NIVS.Open"=FALSE) -> (w331:T2)
                  }
                }
              }
              frame Error {
              }
            }
          }
          frame "NIVS.GetChannels" {
            # "Use the page names to group the alias channels and waveform channels.  Cache the alias paths for future use."
            n126 = call "NIVS.FilterChannels.vi"("error in (no error)"=w339, "Cluster in"=w338) -> ("error out"=w337:errorcluster, "Cluster out"=w336:T2)  [unwired: 8 in]
          }
          frame "NIVS.Read" {
            # "Read non waveform channels from VeriStand.  Format the data and update the table."
            n127 = call "NIVS.Channels.Read.vi"("error in (no error)"=w341, "State Variables"=w342) -> ("error out"=w340:errorcluster)  [unwired: 9 in]
          }
          frame "Page.Back" {
            # "Go back one page."
            n128 = call "Page.Back.vi"("error in (no error)"=w345, "State Variables"=w344) -> ("error out"=w346:errorcluster, "State Variables"=w343:T2)  [unwired: 8 in]
          }
          frame "Page.Next" {
            # "Go forward one page."
            n129 = call "Page.Next.vi"("error in (no error)"=w349, "State Variables"=w348) -> ("error out"=w350:errorcluster, "State Variables"=w347:T2)  [unwired: 8 in]
          }
          frame "Page.Publish" {
            # "Publish the current page selection to the main application."
            n130 = Unbundle By Name(w362) -> ("Station.ID"=w361:string, "UI.Pages"=w355:T1[], "Page.Index"=w354:u32)
            n131 = Index Array(array=w355, index=w354) -> (element=w353:T1)
            n132 = Unbundle By Name(w353) -> ("Name"=w352:string)
            n133 = Concatenate Strings(w361, "\\" ("string"), w352) -> (w359:string)
            n134 = call <vilib>:"Send Local Message.vi"("receiver process (\"\" - local)"="MainExecutionTool" ("string"), "message name"="Page.Published" ("string"), "message value"=w359, "error in"=w351) -> ("error out"=w356:errorcluster)  [unwired: 9 in, 2 out]
            n135 = call <vilib>:"Clear Errors.vi"("error in (no error)"=w356) -> ()  [unwired: 5 in, 2 out]
          }
          frame "Pages.Publish" {
            # "Publish all the found pages to the main application."
            n136 = Unbundle By Name(w375) -> ("Station.ID"=w363:string, "UI.Pages"=w371:T1[], "NIVS.Deployed"=w370:bool)
            n137 = case shown="False" w370 {
              tunnel: w371 -> [_ w378]
              tunnel: [string[] [] w377] -> w366
              frame False {
              }
              frame True {
                n138 = for {
                  tunnel: w378 -> [w381] mode=indexing
                  tunnel: [w380] -> w377 mode=indexing if=w379
                  n139 = Unbundle By Name(w381) -> ("Name"=w380:string, "Found?"=w379:bool)
                }
              }
            }
            n140 = Bundle By Name(cluster=cluster{"Station.ID":string, "Pages":string[]} {"Station.ID"="", "Pages"=[]}, "Station.ID"=w363, "Pages"=w366) -> (w365:cluster{"Station.ID":string, "Pages":string[]})
            n141 = Flatten To String(anything=w365, error in (no error)=w369) -> (data string=w364:string, error out=w368:errorcluster)  [unwired: 2 in, 1 out]
            n142 = call <vilib>:"Send Local Message.vi"("receiver process (\"\" - local)"="MainExecutionTool" ("string"), "message name"="Pages.Published" ("string"), "message value"=w364) -> ("error out"=w372:errorcluster)  [unwired: 10 in, 2 out]
            n143 = call <vilib>:"Clear Errors.vi"("error in (no error)"=w372) -> ()  [unwired: 5 in, 2 out]
          }
          frame "Page.Set" {
            # "Main application has commanded to change the current page.  Handle accordingly."
            n144 = call <vilib>:"Send Local Messages.vi"("message queue in"=w386, "message names"=string[] ["UI.ClearTable", "NIVS.Read", "Tab.Set"], "error in"=w388) -> ("message queue out"=w385:T13, "error out"=w387:errorcluster)  [unwired: 10 in, 1 out]
            n145 = Unbundle By Name(w383) -> ("UI.Displays"=w395:refnum<vi>)
            n146 = property class="TabCtl"(reference=w395, error in=w387) -> (error out=w393:errorcluster, "Value"=w391:variant)  [unwired: 1 out]
            n147 = local read "Displays"() -> (w389:enum32{"Default", "OSCOPE"})
            n148 = Variant To Data(error in=w393, type=w389, Variant=w391) -> (data=w390:enum32{"Default", "OSCOPE"}, error out=w392:errorcluster)
            n149 = case shown="\"OSCOPE\"" w390 {
              tunnel: w392 -> [w398 w401]
              tunnel: [w398 w400] -> w394
              tunnel: w385 -> [_ w399]
              frame Default {
                # "Do nothing."
              }
              frame "OSCOPE" {
                # "OSCOPE is the current page.  Close the waveform references and re-initialize the graph/group."
                n150 = call <vilib>:"Send Local Messages.vi"("message queue in"=w399, "message names"=string[] ["Waveforms.Close", "UI.ClearGraph", "UI.ChangeGroup"], "error in"=w401) -> ("error out"=w400:errorcluster)  [unwired: 10 in, 2 out]
              }
            }
            n151 = call "Page.Set.vi"("error in (no error)"=w394, "message value"=w397, "State Variables"=w383) -> ("error out"=w396:errorcluster, "State Variables"=w382:T2)  [unwired: 7 in]
          }
          frame "Tab.Set" {
            # "Change the view to a new tab. Set GUI and table to appropriate structures."
            n152 = call "Tab.Set.vi"("error in (no error)"=w405, "State Variables"=w404) -> ("error out"=w406:errorcluster, "State Variables out"=w403:T2)  [unwired: 8 in]
          }
          frame "UI.Open" {
            # "Open the front panel."
            n153 = invoke class="VI" method="FP.Open"(error in=w408) -> (error out=w407:errorcluster)  [unwired: 4 in, 4 out]
          }
          frame "UI.Close" {
            # "Close the front panel."
            n154 = flat-sequence {
              tunnel: [w414] -> w410
              tunnel: w411 -> [w414]
              tunnel: [w413] -> _
              frame #0 {
                n155 = invoke class="VI" method="FP.Close"() -> (error out=w413:errorcluster)  [unwired: 3 in, 2 out]
                n156 = Wait (ms)(milliseconds to wait=u32 500) -> ()  [unwired: 1 out]
              }
            }
          }
          frame "UI.SetBusy" {
            # "Set the cursor to busy by queueing command to main application."
            n157 = call <vilib>:"Send Local Message.vi"("receiver process (\"\" - local)"="MainExecutionTool" ("string"), "message name"=w416, "error in"=w417) -> ("error out"=w418:errorcluster)  [unwired: 10 in, 2 out]
            n158 = call <vilib>:"Clear Errors.vi"("error in (no error)"=w418) -> ()  [unwired: 5 in, 2 out]
            n159 = call <vilib>:"Set Busy.vi"() -> ()  [unwired: 10 in, 2 out]
          }
          frame "UI.UnsetBusy" {
            # "Release the cursor from busy by queueing command to main application."
            n160 = call <vilib>:"Send Local Message.vi"("receiver process (\"\" - local)"="MainExecutionTool" ("string"), "message name"=w422, "error in"=w421) -> ("error out"=w423:errorcluster)  [unwired: 10 in, 2 out]
            n161 = call <vilib>:"Clear Errors.vi"("error in (no error)"=w423) -> ()  [unwired: 5 in, 2 out]
            n162 = call <vilib>:"Unset Busy.vi"() -> ()  [unwired: 11 in, 1 out]
          }
          frame "UI.Update" {
            # "Show or hide the GUI to the user."
            n163 = Unbundle By Name(w433) -> ("UI.ToolTab"=w432:refnum<vi>, "NIVS.Deployed"=w431:bool)
            n164 = Select(t=enum32{"Enable", "Disable"}."Enable" ("Value"), s=w431, f=enum32{"Enable", "Disable"}."Disable") -> (s? t:f=w428:enum32{"Enable", "Disable"})
            n165 = property class="TabCtl (strict)"(reference=w432, error in=w427, "Value"=w428) -> (error out=w426:errorcluster)  [unwired: 1 out]
          }
          frame "UI.ChangeGroup" {
            # "Reset the groups to zero."
            n166 = Unbundle By Name(w438) -> ("Waveform.Groups"=w437:refnum<vi>)
            n167 = property class="Ring (strict)"(reference=w437, error in=w436, "Value"=u8 0) -> (error out=w435:errorcluster)  [unwired: 1 out]
          }
          frame "UI.UpdateGroups" {
            # "Load the waveform groups ring with the available options."
            n168 = call "NIVS.Waveforms.Group.vi"("error in (no error)"=w440, "Cluster"=w441) -> ("error out"=w439:errorcluster)  [unwired: 9 in]
          }
          frame "UI.ClearTable" {
            # "Re-initialize the table."
            n169 = call "Table.Clear.vi"("error in (no error)"=w443, "State Variables"=w444) -> ("error out"=w442:errorcluster)  [unwired: 9 in]
          }
          frame "UI.ClearGraph" {
            # "Re-initialize the graph."
            n170 = Unbundle By Name(w447) -> ("Waveform.Graph"=w455:refnum<vi>, "Waveform.Legend"=w448:T3)
            n171 = invoke class="WFGraph (strict)" method="Reinit To Default"(reference=w455, error in=w453) -> (reference out=w454:refnum<vi>, error out=w452:errorcluster)  [unwired: 1 in, 1 out]
            n172 = Bundle By Name(cluster=w447, "Waveforms.Size"=1) -> (w446:T2)
            n173 = property class="WFGraph (strict)"(reference=w454, error in=w452, "Value"=waveform(dbl)[] [{"t0"=timestamp(0 s since 1904-01-01), "dt"=1.0, "Y"=[]}], "LegNumRows"=u32 1 ("Legend:Number of Rows"), "Active Plot"=u32 0, "Plot.Plot Name"="Plot 0", "LegScrollPos"=u32 0 ("Legend:Scroll Position"), "LegScrollVis"=FALSE ("Legend:Scrollbar Visible"), "LegPos"=w448) -> (error out=w458:errorcluster)  [unwired: 1 out]
          }
          frame "UI.ClearGroups" {
            # "Re-initialize the waveform groups ring."
            n174 = Unbundle By Name(w465) -> ("Waveform.Groups"=w464:refnum<vi>)
            n175 = property class="Ring (strict)"(reference=w464, error in=w463, "Strings []"=string[] [], "Value"=u8 0) -> (error out=w462:errorcluster)  [unwired: 1 out]
          }
          frame "Waveforms.Init" {
            # "Open references and events for the VS waveforms and re-initialize the graph legend and display."
            n176 = call "Waveforms.Start.vi"("error in (no error)"=w466, "Cluster in"=w468) -> ("error out"=w469:errorcluster, "Cluster out"=w467:T2)  [unwired: 8 in]
          }
          frame "Waveforms.SelectAll" {
            # "Enable all the channels on the graph."
            n177 = Unbundle By Name(w482) -> ("Waveforms.Size"=w470:i32, "Waveform.Graph"=w471:refnum<vi>, "VI.Ref"=w481:refnum<vi>)
            n178 = property class="VI"(reference=w481, error in=w478) -> (error out=w479:errorcluster, "Panel"=w480:refnum<vi>)  [unwired: 1 out]
            n179 = property class="Pnl"(reference=w480, error in=w479, "DeferPanUpdts"=TRUE ("Defer Panel Updates")) -> (reference out=w474:refnum<vi>, error out=w472:errorcluster)
            n180 = for {
              N: w470 -> [_]
              tunnel: w471 -> [w491]
              shift-right: [w487] -> w475
              shift-left: w472 -> [w490]
              i -> [w489]
              n181 = property class="WFGraph (strict)"(reference=w491, error in=w490, "Active Plot"=w489, "Plot.Visible?"=TRUE ("Legend:Visible")) -> (error out=w487:errorcluster)  [unwired: 1 out]
            }
            n182 = flat-sequence {
              tunnel: [w486] -> w476
              tunnel: w475 -> [w486]
              tunnel: w474 -> [w485]
              tunnel: FALSE ("Defer Panel Updates") -> [w484]
              tunnel: [w483] -> _
              frame #0 {
                n183 = property class="Pnl"(reference=w485, "DeferPanUpdts"=w484) -> (error out=w483:errorcluster)  [unwired: 1 in, 1 out]
              }
            }
          }
          frame "Waveforms.DeselectAll" {
            # "Disable all the channels on the graph."
            n184 = Unbundle By Name(w504) -> ("Waveforms.Size"=w494:i32, "Waveform.Graph"=w492:refnum<vi>, "VI.Ref"=w503:refnum<vi>)
            n185 = property class="VI"(reference=w503, error in=w500) -> (error out=w501:errorcluster, "Panel"=w502:refnum<vi>)  [unwired: 1 out]
            n186 = property class="Pnl"(reference=w502, error in=w501, "DeferPanUpdts"=TRUE ("Defer Panel Updates")) -> (reference out=w496:refnum<vi>, error out=w493:errorcluster)
            n187 = for {
              N: w494 -> [_]
              tunnel: w492 -> [w513]
              shift-right: [w509] -> w497
              shift-left: w493 -> [w512]
              i -> [w511]
              n188 = property class="WFGraph (strict)"(reference=w513, error in=w512, "Active Plot"=w511, "Plot.Visible?"=FALSE ("Legend:Visible")) -> (error out=w509:errorcluster)  [unwired: 1 out]
            }
            n189 = flat-sequence {
              tunnel: [w508] -> w498
              tunnel: w497 -> [w508]
              tunnel: w496 -> [w507]
              tunnel: FALSE ("Defer Panel Updates") -> [w506]
              tunnel: [w505] -> _
              frame #0 {
                n190 = property class="Pnl"(reference=w507, "DeferPanUpdts"=w506) -> (error out=w505:errorcluster)  [unwired: 1 in, 1 out]
              }
            }
          }
          frame "Waveforms.Close" {
            # "Close all the VS waveform references and events."
            n191 = Unbundle By Name(w516) -> ("Waveforms"=w518:T18)
            n192 = flat-sequence {
              tunnel: w519 -> [w520]
              tunnel: [w522] -> _
              tunnel: w518 -> [w521]
              tunnel: [w520] -> w514
              frame #0 {
                n193 = call "Waveforms.Close.vi"("error in (no error)"=w520, "Waveforms"=w521) -> ("error out"=w522:errorcluster)  [unwired: 9 in]
              }
            }
            n194 = Bundle By Name(cluster=w516, "Waveforms"=T14 {"Waveform.Refs"=[], "WaveformStreaming.Event.Refs"={"Callback Refnum"=refnum, "Data Event"=refnum, "Event Refnum"=refnum, "WaveformDataWatcherDBL"=refnum}, "WaveformStreaming.Ref"=refnum} ("Waveforms.Refs")) -> (w515:T2)
          }
          frame Default {
          }
        }
      }
    }
    frame Error {
      n195 = disable-structure shown="Enabled" {
        frame Enabled {
          n196 = invoke class="VI" method="FP.Close"() -> ()  [unwired: 3 in, 3 out]
        }
        frame Disabled {
        }
      }
    }
  }
  "Station ID" <- "Station.ID"
